vi "Write This VI.vi"(8 "error in (no error)":errorcluster, 10 "This VI":refnum<vi>, 11 "UI in":refnum<class "UI.lvclass">) -> (0 "error out":errorcluster, 3 "UI out":refnum<class "UI.lvclass">)   [LabVIEW 2017, in "Generic UI Actor.lvlib" / "UI.lvclass"]
uses:
  UI.lvclass
  UI.lvclass/UI.ctl
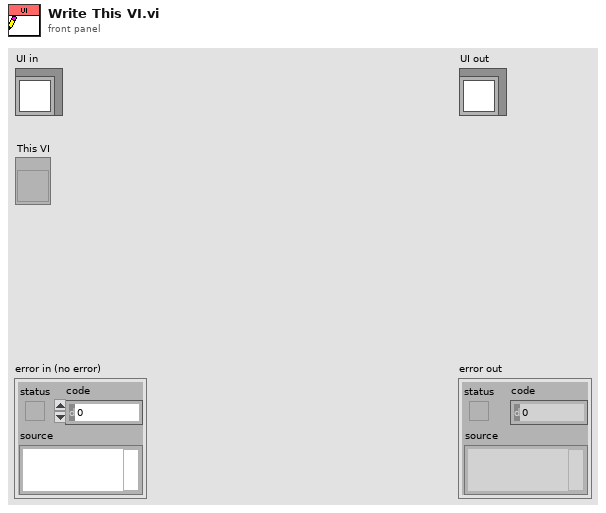
[diagram p1: front panel]
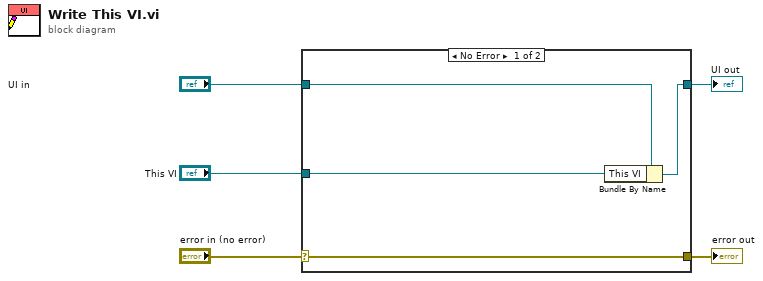
[diagram p0: block diagram]
diagram:
  n1 = case shown="No Error" "error in (no error)" {
    selector: "error in (no error)" -> [w9 w10]
    tunnel: [w9 w10] -> w4
    tunnel: [w7 w11] -> w2
    tunnel: "UI in" -> [w8 w11]
    tunnel: "This VI" -> [w6 _]
    frame No Error {
      n2 = Bundle By Name(cluster=w8, "This VI"=w6) -> (w7:refnum<class "UI.lvclass">)
    }
    frame Error {
    }
  }
  "error out" <- w4
  "UI out" <- w2
